vi "Align & Distribute UI.vi"() -> (0 "Distribute Type valid?":bool, 1 "Align Type valid?":bool, 2 "Distribute Type":T11(ring), 3 "Align Type":T12(ring))   [LabVIEW 2017, in "Align and Distribute.lvlib"]
uses:
  Align and Distribute.lvlib
  Align Objects.ctl
  Dist Top Edges.ctl
  Dist Bottom Edges.ctl
  Dist Vertical Gap.ctl
  Dist Vertical Compress.ctl
  Dist Left Edges.ctl
  Dist Horizontal Centers.ctl
  Dist Right Edges.ctl
  Dist Horizontal Gap.ctl
  Dist Horizontal Compress.ctl
  Distribute Objects.ctl
panel:
  out "Label":string
  in  "Distribute Objects":T1
  in  "Align Objects":T13
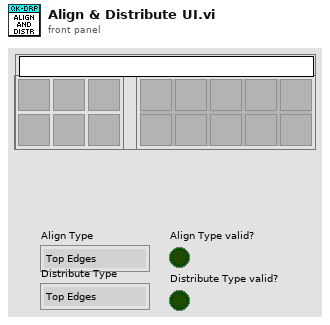
[diagram p1: front panel]
types:
  T1 = typedef "Align and Distribute.lvlib/Distribute Objects.ctl" = cluster{"Top Edges":T2, "Vertical Centers":bool, "Bottom Edges":T3, "Vertical Gap":T4, "Vertical Compress":T5, "Left Edges":T6, "Horizontal Centers":T7, "Right Edges":T8, "Horizontal Gap":T9, "Horizontal Compress":T10}
  T2 = typedef "Align and Distribute.lvlib/Dist Top Edges.ctl" = bool
  T3 = typedef "Align and Distribute.lvlib/Dist Bottom Edges.ctl" = bool
  T4 = typedef "Align and Distribute.lvlib/Dist Vertical Gap.ctl" = bool
  T5 = typedef "Align and Distribute.lvlib/Dist Vertical Compress.ctl" = bool
  T6 = typedef "Align and Distribute.lvlib/Dist Left Edges.ctl" = bool
  T7 = typedef "Align and Distribute.lvlib/Dist Horizontal Centers.ctl" = bool
  T8 = typedef "Align and Distribute.lvlib/Dist Right Edges.ctl" = bool
  T9 = typedef "Align and Distribute.lvlib/Dist Horizontal Gap.ctl" = bool
  T10 = typedef "Align and Distribute.lvlib/Dist Horizontal Compress.ctl" = bool
  T11 = enum32{"Top Edges", "Vertical Centers", "Bottom Edges", "Vertical Gap", "Vertical Compress", "Left Edges", "Horizontal Centers", "Right Edges", "Horizontal Gap", "Horizontal Compress"}
  T12 = enum32{"Top Edges", "Vertical Centers", "Bottom Edges", "Left Edges", "Horizontal Centers", "Right Edges"}
  T13 = typedef "Align and Distribute.lvlib/Align Objects.ctl" = cluster{"Top Edges":bool, "Vertical Centers":bool, "Bottom Edges":bool, "Left Edges":bool, "Horizontal Centers":bool, "Right Edges":bool}
  T14 = typedef "eventvkey.ctl" = enum16{"ASCII", "Enter", "Return", "Shift", "Ctrl", "Alt", "Cmd", "Opt", "Caps", "NumLock", "Clear", "Break", "Up", "Down", "Left", "Right", "Insert", "Delete", "Home", "End", "PageUp", "PageDown", "Escape", "Help", "Pause", "ScrollLock", "F1", "F2", "F3", "F4", "F5", "F6", "F7", "F8", "F9", "F10", "F11", "F12", "F13", "F14", "F15", "F16", "F17", "F18", "F19", "F20", "F21", "F22", "F23", "F24", "Play", "VolumeUp", "VolumeDown", "Mute", "Two Byte Char"}
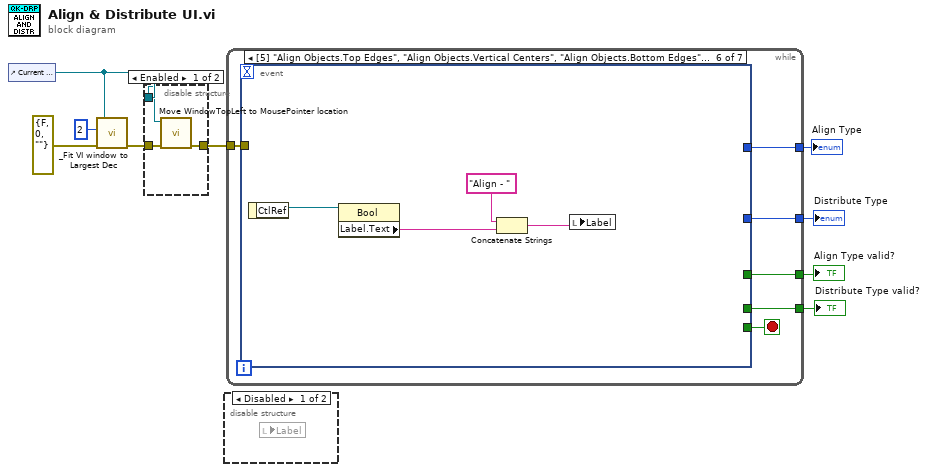
[diagram p0: block diagram]
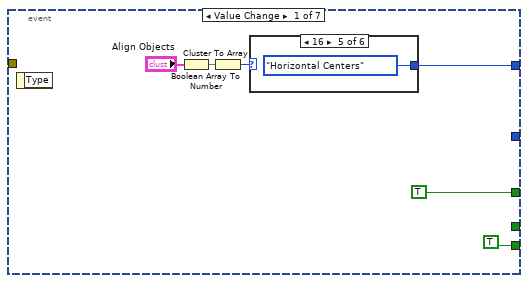
[diagram p4: hidden frame]
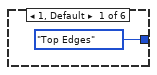
[diagram p5: hidden frame]
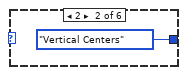
[diagram p6: hidden frame]
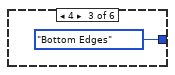
[diagram p7: hidden frame]
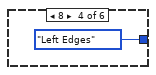
[diagram p8: hidden frame]
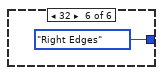
[diagram p9: hidden frame]
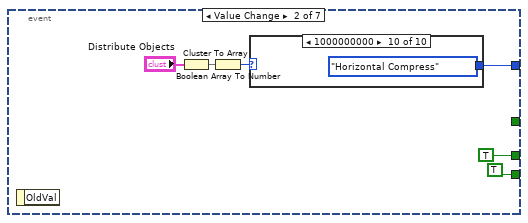
[diagram p10: hidden frame]
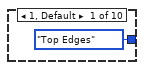
[diagram p11: hidden frame]
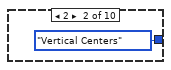
[diagram p12: hidden frame]
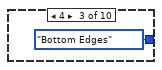
[diagram p13: hidden frame]
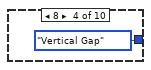
[diagram p14: hidden frame]
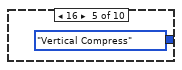
[diagram p15: hidden frame]
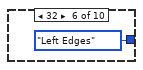
[diagram p16: hidden frame]
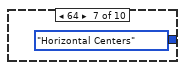
[diagram p17: hidden frame]
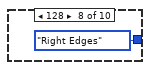
[diagram p18: hidden frame]
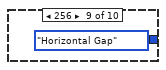
[diagram p19: hidden frame]
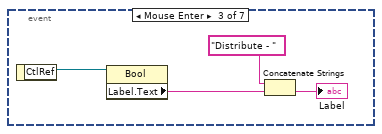
[diagram p20: hidden frame]
diagram:
  n1 = control-ref of="Current VI Reference"() -> (w1:refnum<vi>)
  n2 = call "_Fit VI window to Largest Dec.vi"("error in (no error)"=errorcluster {"status"=FALSE, "code"=0, "source"=""}, "border spacing (2 px)"=2, "VI Ref (calling VI)"=w1) -> ("error out"=w2:errorcluster)  [unwired: 3 in, 1 out]
  n3 = disable-structure shown="Enabled" {
    disable-tunnel: [w12 w13] -> w7
    disable-tunnel: w2 -> [w11 w13]
    disable-tunnel: w1 -> [w10 _]
    frame Enabled {
      n4 = call "Move WindowTopLeft to MousePointer location.vi"("error in (no error)"=w11, "VIRef"=w10) -> ("error out"=w12:errorcluster)  [unwired: 9 in]
    }
    frame Disabled {
    }
  }
  n5 = disable-structure shown="Disabled" {
    frame Disabled {
      n6 = local read "Label"() -> ()  [unwired: 1 in]
    }
    frame Enabled {
    }
  }
  n7 = while {
    tunnel: [w19] -> w9
    tunnel: [w18] -> w8
    tunnel: w7 -> [w17]
    tunnel: [w16] -> w6
    tunnel: [w15] -> w5
    stop <- w14 stop-if-true
    n8 = event shown="[5] \"Align Objects.Top Edges\", \"Align Objects.Vertical Centers\", \"Align Objects.Bottom Edges\", \"Align Objects.Left Edges\", \"Align Objects.Horizontal Centers\", \"Align Objects.Right Edges\": Mouse Enter" {
      selector: _ -> [_ _ _ _ _ _ _]
      dyn-events: _ -> [_ _ _ _ _ _ _]
      timeout: _ -> [_ _ _ _ _ _ _]
      tunnel: [w22 _ _ _ _ _ w64] -> w19
      tunnel: [_ w34 _ _ _ _ w63] -> w18
      tunnel: w17 -> [_ _ _ _ _ _ _]
      tunnel: [TRUE _ _ _ _ _ w60] -> w16
      tunnel: [_ TRUE _ _ _ _ w59] -> w15
      tunnel: [TRUE TRUE _ _ _ _ w58] -> w14
      event Value Change {
        n9 = event-data() -> ()  [unwired: 1 in, 1 out]
        n10 = Cluster To Array(cluster="Align Objects") -> (array=w24:bool[])
        n11 = Boolean Array To Number(Boolean array=w24) -> (number=w23:u32)
        n12 = case shown="16" w23 {
          tunnel: [T12."Top Edges" ("Align Type") T12."Vertical Centers" ("Align Type") T12."Bottom Edges" ("Align Type") T12."Left Edges" ("Align Type") T12."Horizontal Centers" ("Align Type") T12."Right Edges" ("Align Type")] -> w22
          frame 1, Default {
          }
          frame 2 {
          }
          frame 4 {
          }
          frame 8 {
          }
          frame 16 {
          }
          frame 32 {
          }
        }
      }
      event Value Change {
        n13 = event-data() -> ()  [unwired: 1 in, 1 out]
        n14 = Cluster To Array(cluster="Distribute Objects") -> (array=w35:T10[])
        n15 = Boolean Array To Number(Boolean array=w35) -> (number=w36:u32)
        n16 = case shown="1000000000" w36 {
          tunnel: [T11."Top Edges" ("DistributeType") T11."Vertical Centers" ("DistributeType") T11."Bottom Edges" ("DistributeType") T11."Vertical Gap" ("DistributeType") T11."Vertical Compress" ("DistributeType") T11."Left Edges" ("DistributeType") T11."Horizontal Centers" ("DistributeType") T11."Right Edges" ("DistributeType") T11."Horizontal Gap" ("DistributeType") T11."Horizontal Compress" ("DistributeType")] -> w34
          frame 1, Default {
          }
          frame 2 {
          }
          frame 4 {
          }
          frame 8 {
          }
          frame 16 {
          }
          frame 32 {
          }
          frame 64 {
          }
          frame 128 {
          }
          frame 256 {
          }
          frame 512 {
          }
        }
      }
      event Mouse Enter {
        n17 = event-data() -> ("CtlRef"=w51:refnum<vi>)  [unwired: 1 in]
        n18 = property class="Bool"(reference=w51) -> ("Label.Text"=w50:string)  [unwired: 1 in, 2 out]
        n19 = Concatenate Strings("Distribute - " ("string"), w50) -> (→"Label":string)
      }
      event Mouse Leave {
        n20 = event-data() -> ()  [unwired: 1 in, 1 out]
        n21 = local write "Label"("" ("Label")) -> ()
      }
      event Mouse Leave {
        n22 = event-data() -> ()  [unwired: 1 in, 4 out]
        n23 = local write "Label"("" ("Label")) -> ()
      }
      event Mouse Enter {
        n24 = event-data() -> ("CtlRef"=w57:refnum<vi>)  [unwired: 1 in]
        n25 = property class="Bool"(reference=w57) -> ("Label.Text"=w56:string)  [unwired: 1 in, 2 out]
        n26 = Concatenate Strings("Align - " ("string"), w56) -> (w54:string)
        n27 = local write "Label"(w54) -> ()
      }
      event Key Down {
        n28 = event-data() -> ("Char"=w65:i16, "VKey"=w61:T14)  [unwired: 1 in]
        n29 = To Unsigned Byte Integer(number=w65) -> (unsigned 8bit integer=w66:u8)
        n30 = Build Array(w66) -> (w67:u8[])
        n31 = Byte Array To String(unsigned byte array=w67) -> (string=w62:string)
        n32 = case shown="\"Escape\"" w61 {
          tunnel: [w72 _] -> w64
          tunnel: [w71 _] -> w63
          tunnel: w62 -> [w70 _]
          tunnel: [FALSE _] -> w60
          tunnel: [FALSE _] -> w59
          tunnel: [_ TRUE] -> w58
          frame "ASCII", Default {
            n33 = case shown="\"L\", \"l\", Default" w70 {
              tunnel: [T11."Vertical Compress" ("DistributeType") T11."Vertical Compress" ("DistributeType") T11."Horizontal Compress" ("DistributeType") T11."Horizontal Compress" ("DistributeType") T11."Horizontal Compress" ("DistributeType") T11."Vertical Compress" ("DistributeType")] -> w71
              frame "R", "r" {
              }
              frame "L", "l", Default {
              }
              frame "T", "t" {
              }
              frame "B", "b" {
              }
              frame "V", "v" {
              }
              frame "H", "h" {
              }
            }
            n34 = case shown="\"V\", \"v\"" w70 {
              tunnel: [T12."Right Edges" ("Align Type") T12."Left Edges" ("Align Type") T12."Top Edges" ("Align Type") T12."Bottom Edges" ("Align Type") T12."Vertical Centers" ("Align Type") T12."Horizontal Centers" ("Align Type")] -> w72
              frame "R", "r" {
              }
              frame "L", "l", Default {
              }
              frame "T", "t" {
              }
              frame "B", "b" {
              }
              frame "V", "v" {
              }
              frame "H", "h" {
              }
            }
          }
          frame "Escape" {
          }
        }
      }
    }
  }
  "Align Type" <- w9
  "Distribute Type" <- w8
  "Align Type valid?" <- w6
  "Distribute Type valid?" <- w5
